vi "ColorDetect2.0.vi"(0 "new picture":picture, 5 "Color 1 Lower":u32(colorbox), 7 "Color 1 Upper":u32(colorbox), 11 "error in (no error)":errorcluster) -> (4 "out picture":picture, 6 "image":u8[][](array[numeric]), 8 "found":u32[][](array[numeric]), 15 "error out":errorcluster)   [LabVIEW 2014, in "QwaveSys Raspberry Pi Library.lvlib"]
uses:
  QwaveSys Raspberry Pi Library.lvlib
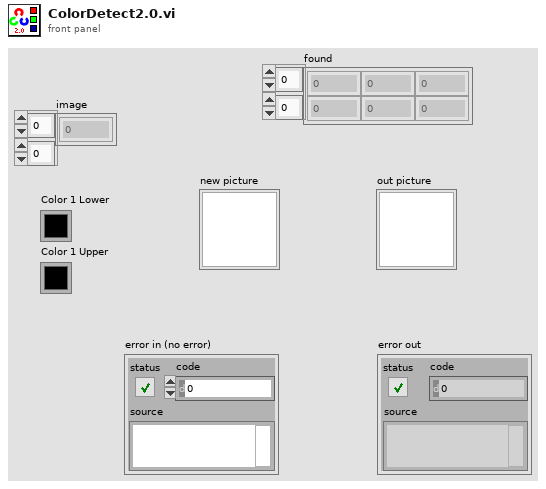
[diagram p1: front panel]
types:
  T1 = cluster{"Width":u16, "Style":enum32{"Solid", "Dash", "Dot", "DashDot", "DashDotDot"}}
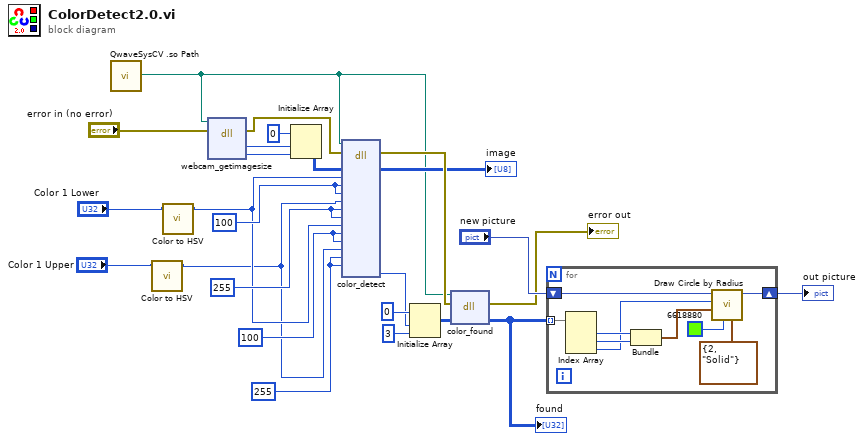
[diagram p0: block diagram]
diagram:
  w11 = u8 100
  w10 = u8 255
  w12 = u8 255
  w13 = u8 100
  n1 = call "QwaveSysCV .so Path.vi"() -> ("QwaveSys .so Path"=w5:path)  [unwired: 5 in]
  n2 = call "Color to HSV.vi"("Color Box"="Color 1 Upper") -> ("Hue (0-180)"=w1:u8)  [unwired: 8 in, 2 out]
  n3 = call "Color to HSV.vi"("Color Box"="Color 1 Lower") -> ("Hue (0-180)"=w3:u8)  [unwired: 8 in, 2 out]
  n4 = dll-call lib="libqwavesys.so" fn="webcam_getimagesize"(path in=w5, error in="error in (no error)") -> (error out=w16:errorcluster, "rows"=w24:i32, "cols"=w25:i32)  [unwired: 4 in, 1 out]
  n5 = Initialize Array(u8 0 ("element"), w24, w25) -> (w23:u8[][])
  n6 = dll-call lib="libqwavesys.so" fn="color_detect"(path in=w5, error in=w16, "image"=w23, "Alower_h"=w3, "Alower_s"=w13, "Alower_v"=w13, "Aupper_h"=w1, "Aupper_s"=w12, "Aupper_v"=w12, "Blower_h"=w3, "Blower_s"=w11, "Blower_v"=w11, "Bupper_h"=w1, "Bupper_s"=w10, "Bupper_v"=w10) -> (error out=w15:errorcluster, "image"=→"image":u8[][], "found"=w14:i32)  [unwired: 15 in, 1 out]
  n7 = Initialize Array "Initialize Array"(u32 0 ("element"), w14, 3 ("dimension size")) -> (w19:u32[][])
  n8 = dll-call lib="libqwavesys.so" fn="color_found"(path in=w5, error in=w15, "found"=w19) -> (error out=→"error out":errorcluster, "found"=w18:u32[][])  [unwired: 2 in, 1 out]
  "found" <- w18
  n9 = for {
    tunnel: w18 -> [w32] mode=indexing
    shift-right: [w26] -> w8
    shift-left: "new picture" -> [w27]
    n10 = Index Array(array=w32) -> (element #1=w31:u32, element #2=w30:u32, element #3=w29:u32)  [unwired: 3 in]
    n11 = Bundle(w31, w30) -> (w34:cluster{u32, u32})  [unwired: 1 in]
    n12 = call <vilib>:"Draw Circle by Radius.vi"("pen"=T1 {"Width"=2, "Style"=enum."Solid"}, "color(black)"=u32 6618880, "pixel center"=w34, "radius"=w29, "picture"=w27) -> ("new picture"=w26:picture)  [unwired: 6 in]
  }
  "out picture" <- w8
